vi "GE5565 Set DMA RW (Cluster) mod.vi"(4 "error in (no error)":errorcluster, 5 "operation (read)":enum16{"read", "write"}(ring), 7 "VMIC-5565":T1) -> (0 "error out":errorcluster, 3 "VMIC-5565":T1)   [LabVIEW 2017, in "GE_RM_Real Time.lvlib"]
uses:
  <vilib>/Instr/_visa.llb/VISA Register Access Address Space.ctl
  GE_RM_Real Time.lvlib
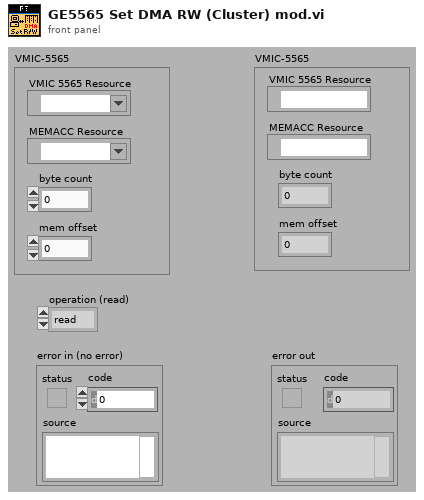
[diagram p1: front panel]
types:
  T1 = cluster{"VMIC 5565 Resource":refnum<visa-resource-name>, "MEMACC Resource":refnum<visa-resource-name>, "byte count":u32, "mem offset":u32}
  T2 = typedef "VISA Register Access Address Space.ctl" = u16
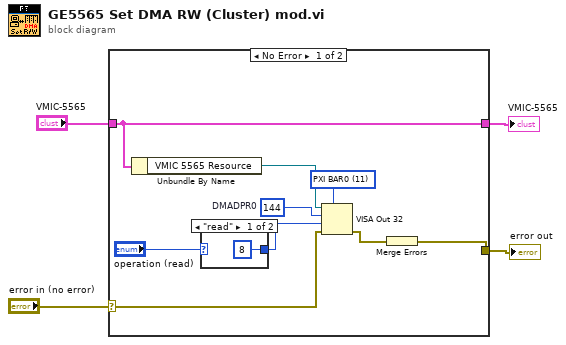
[diagram p0: block diagram]
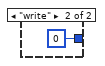
[diagram p2: hidden frame]
diagram:
  n1 = case shown="No Error" "error in (no error)" {
    selector: "error in (no error)" -> [w8 w16]
    tunnel: "VMIC-5565" -> [w6 w17]
    tunnel: [w6 w17] -> w1
    tunnel: [w9 w16] -> w3
    frame No Error {
      w5 = T2 11 items=["VXI/VME A16"=1, "VXI/VME A24"=2, "VXI/VME A32"=3, "VXI/VME A64"=4, "PXI Memory Allocations"=9, "PXI Configuration"=10, "PXI BAR0"=11, "PXI BAR1"=12, "PXI BAR2"=13, "PXI BAR3"=14, "PXI BAR4"=15, "PXI BAR5"=16] ("Address Space")
      w12 = u32 144  # DMADPR0
      n2 = Unbundle By Name(w6) -> ("VMIC 5565 Resource"=w7:refnum<visa-resource-name>)
      n3 = case shown="\"read\"" "operation (read)" {
        tunnel: [u32 8 ("value (0)") u32 0 ("value (0)")] -> w11
        frame "read" {
        }
        frame "write" {
        }
      }
      n4 = VISA Out 32(7:w5, 8:w8, 9:w11, 10:w12, 11:w7) -> (0:w10:errorcluster)  [unwired: 1 out]
      n5 = Merge Errors(w10) -> (w9:errorcluster)
    }
    frame Error {
    }
  }
  "error out" <- w3
  "VMIC-5565" <- w1
